vi "Generator.vi"() -> ()   [LabVIEW 2021]
uses:
  <vilib>/Utility/miscctls.llb/LV3DPointTypeDef.ctl
  <vilib>/picture/3D Picture Control/Object/Create Object (drawable).vi
  <vilib>/picture/3D Picture Control/Object/Add Object (no reference).vi
  <vilib>/picture/3D Picture Control/NI_3D Picture Control.lvlib
panel:
  in  "stop":bool
  out "Ball 2 Position":T1
  out "Ball 1 Position":T1
  out "Arm Base Position":T1
  in  "Z axis deg":sgl(slide) min=0 max=360 step=1 scale=0.0..360.0
  in  "Y axis deg":sgl(slide) min=0 max=360 step=1 scale=0.0..360.0
  in  "X Axis Degrees":sgl(slide) min=0 max=360 step=1 scale=0.0..360.0
  in  "X axis deg":sgl(slide) min=0 max=360 step=1 scale=0.0..360.0
  in  "Wall":dbl(slide)=0.5 min=0.0 max=1.0 step=0.05 scale=0.0..1.0
  in  "Background":u32(colorbox)=5789784
  in  "Axis Color":u32(colorbox)=16448250
  in  "Wall Color":u32(colorbox)=6618880
  in  "Machine Color":u32(colorbox)=16711680
  out "Test Area":refnum<vi>(3d-picture)
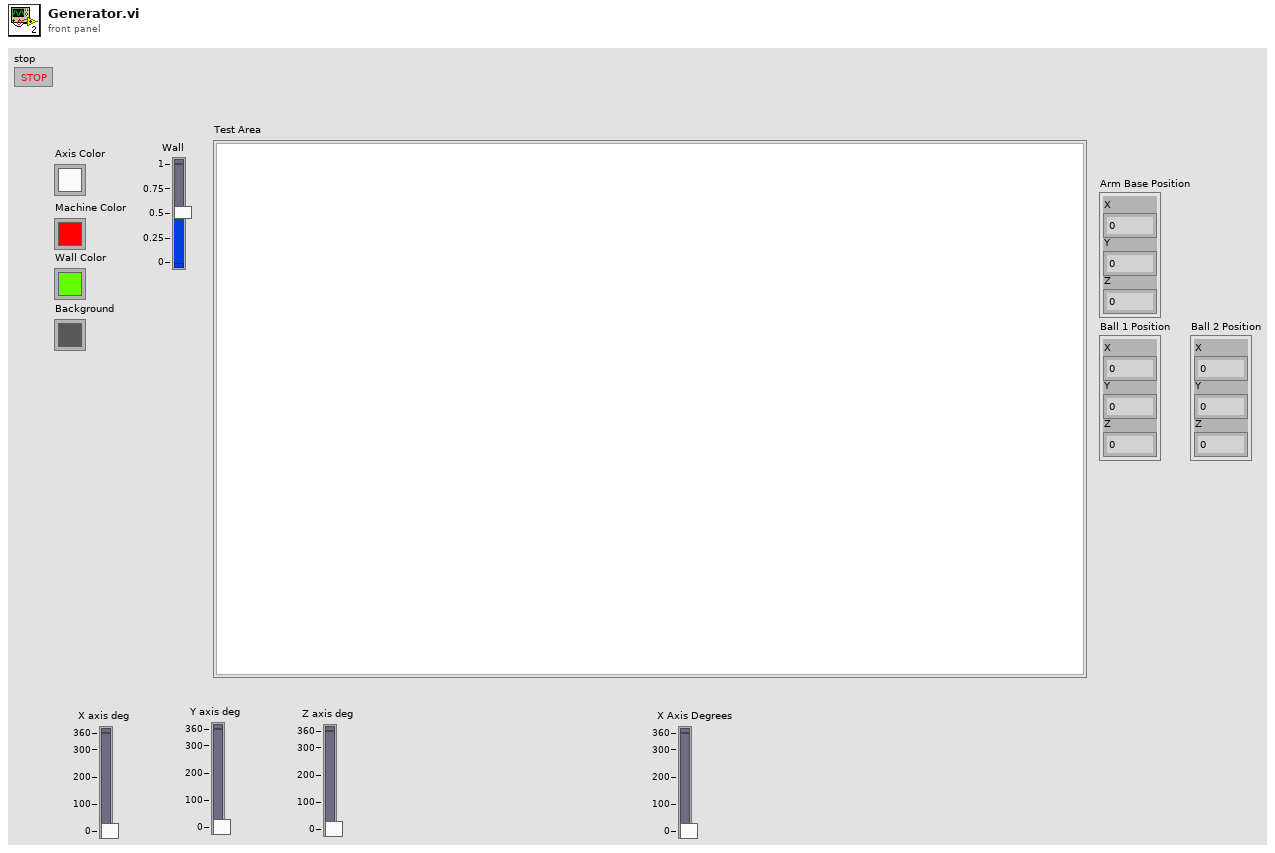
[diagram p1: front panel]
types:
  T1 = typedef "LV3DPointTypeDef.ctl" = cluster{"X":sgl, "Y":sgl, "Z":sgl}
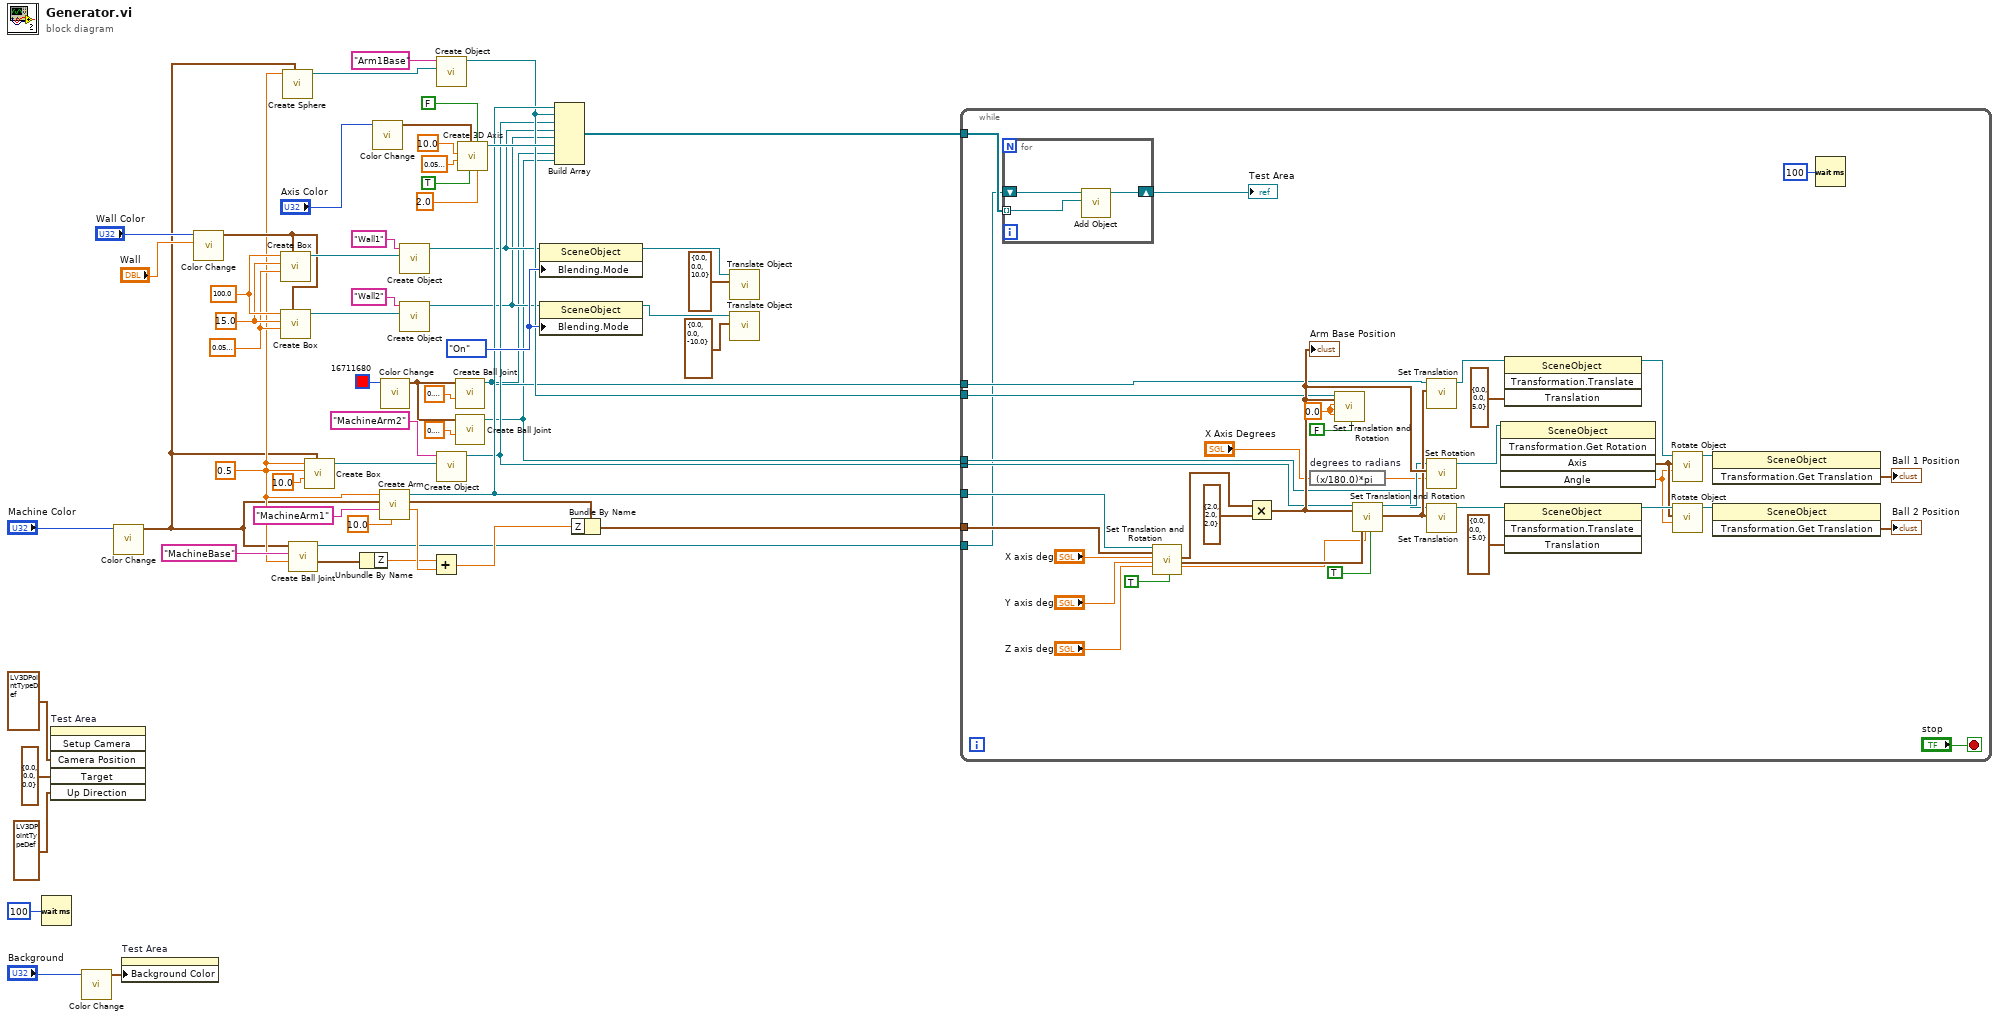
[diagram p0: block diagram]
diagram:
  w17 = sgl 0.5 ("Radius 2")
  w32 = enum16{"Inherit Value", "Off", "On"}."On" ("Blending:Mode")
  w47 = sgl 0.05 ("Length X")
  w48 = sgl 15.0 ("Length X")
  w49 = sgl 100.0 ("Length X")
  n1 = Wait (ms)(milliseconds to wait=u32 100) -> ()  [unwired: 1 out]
  n2 = invoke on="Test Area" class="SceneGraphDisp (strict)" method="Setup Camera"("Camera Position"=T1 {"X"=25.4, "Y"=40.2, "Z"=20.3}, "Target"=T1 {"X"=0.0, "Y"=0.0, "Z"=0.0}, "Up Direction"=T1 {"X"=0.2, "Y"=0.3, "Z"=0.4}) -> ()  [unwired: 3 in, 6 out]
  n3 = call <vilib>:"Color Change.vi"("Color"="Background") -> ("RGBA"=w38:cluster{"R":sgl, "G":sgl, "B":sgl, "A":sgl})  [unwired: 10 in]
  n4 = call <vilib>:"Color Change.vi"("Color"="Machine Color") -> ("RGBA"=w16:cluster{"R":sgl, "G":sgl, "B":sgl, "A":sgl})  [unwired: 10 in]
  n5 = property on="Test Area" class="SceneGraphDisp (strict)"("Background Color"=w38) -> ()  [unwired: 2 in, 2 out]
  n6 = call <vilib>:"Color Change.vi"("Alpha"="Wall", "Color"="Wall Color") -> ("RGBA"=w42:cluster{"R":sgl, "G":sgl, "B":sgl, "A":sgl})  [unwired: 9 in]
  n7 = call <vilib>:"Create Box.vi"("Color"=w42, "Length Z"=w47, "Length Y"=w48, "Length X"=w49) -> ("New Box Refnum"=w50:refnum<vi>)  [unwired: 6 in, 1 out]
  n8 = call <vilib>:"Create Box.vi"("Color"=w42, "Length Z"=w47, "Length Y"=w48, "Length X"=w49) -> ("New Box Refnum"=w34:refnum<vi>)  [unwired: 6 in, 1 out]
  n9 = call <vilib>:"Create Sphere.vi"("Color"=w16, "Radius"=w17) -> ("New Sphere Refnum"=w25:refnum<vi>)  [unwired: 8 in, 1 out]
  n10 = call "Create Ball Joint.vi"("Radius 2"=w17, "Name"="MachineBase", "RGBA"=w16) -> ("Transformation.GetTranslation"=w20:T1, "SceneObject out"=w1:refnum<vi>)  [unwired: 7 in]
  n11 = call <vilib>:"Create Box.vi"("Color"=w16, "Length Z"=sgl 10.0, "Length Y"=w17, "Length X"=w17) -> ("New Box Refnum"=w22:refnum<vi>)  [unwired: 6 in, 1 out]
  n12 = Unbundle By Name(w20) -> ("Z"=w19:sgl)
  n13 = call <vilib>:"Color Change.vi"("Color"="Axis Color") -> ("RGBA"=w40:cluster{"R":sgl, "G":sgl, "B":sgl, "A":sgl})  [unwired: 10 in]
  n14 = call "Create Arm.vi"("Length"=sgl 10.0 ("Length Z"), "Name"="MachineArm1", "Color"=w16, "Radius"=w17) -> ("Half Length"=w26:sgl, "Transformation.GetTranslation"=w30:T1, "SceneObject out"=w9:refnum<vi>)  [unwired: 5 in]
  n15 = call <vilib>:"Color Change.vi"("Color"=u32 16711680) -> ("RGBA"=w12:cluster{"R":sgl, "G":sgl, "B":sgl, "A":sgl})  [unwired: 10 in]
  n16 = call-poly <vilib>:"Create Object.vi"("Geometry"=w50, "Name"="Wall1") -> ("Scene:New Object"=w6:refnum<vi>)  [unwired: 8 in, 1 out]
  n17 = call-poly <vilib>:"Create Object.vi"("Geometry"=w34, "Name"="Wall2") -> ("Scene:New Object"=w5:refnum<vi>)  [unwired: 8 in, 1 out]
  n18 = Add(x=w19, y=w26) -> (x+y=w28:sgl)
  n19 = call-poly <vilib>:"Create Object.vi"("Geometry"=w25, "Name"="Arm1Base") -> ("Scene:New Object"=w8:refnum<vi>)  [unwired: 8 in, 1 out]
  n20 = call-poly <vilib>:"Create Object.vi"("Geometry"=w22, "Name"="MachineArm2") -> ("Scene:New Object"=w7:refnum<vi>)  [unwired: 8 in, 1 out]
  n21 = call "Create Ball Joint.vi"("Radius 2"=sgl 0.6, "RGBA"=w12) -> ("SceneObject out"=w4:refnum<vi>)  [unwired: 8 in, 1 out]
  n22 = call "Create Ball Joint.vi"("Radius 2"=sgl 0.6, "RGBA"=w12) -> ("SceneObject out"=w3:refnum<vi>)  [unwired: 8 in, 1 out]
  n23 = call <vilib>:"Create 3D Axis.vi"("Character Size"=sgl 2.0, "Half plane?"=FALSE, "Axis label?"=TRUE, "Color"=w40, "Radius"=sgl 0.05, "Length"=sgl 10.0) -> ("New Object Refnum"=w10:refnum<vi>)  [unwired: 4 in, 1 out]
  n24 = property class="SceneObject"(reference=w6, "Blending.Mode"=w32) -> (reference out=w35:refnum<vi>)  [unwired: 1 in, 1 out]
  n25 = property class="SceneObject"(reference=w5, "Blending.Mode"=w32) -> (reference out=w33:refnum<vi>)  [unwired: 1 in, 1 out]
  n26 = Build Array(w9, w8, w7, w6, w5, w10, w4, w3) -> (w2:refnum<vi>[])
  n27 = Bundle By Name(cluster=w30, "Z"=w28) -> (w29:T1)
  n28 = call <vilib>:"Translate Object.vi"("Translation"=cluster{"X":sgl, "Y":sgl, "Z":sgl} {"X"=0.0, "Y"=0.0, "Z"=10.0}, "Scene.Object In"=w35) -> ()  [unwired: 8 in, 2 out]
  n29 = call <vilib>:"Translate Object.vi"("Translation"=cluster{"X":sgl, "Y":sgl, "Z":sgl} {"X"=0.0, "Y"=0.0, "Z"=-10.0}, "Scene.Object In"=w33) -> ()  [unwired: 8 in, 2 out]
  n30 = while {
    tunnel: w29 -> [w99]
    tunnel: w9 -> [w69]
    tunnel: w8 -> [w68]
    tunnel: w7 -> [w67]
    tunnel: w4 -> [w66]
    tunnel: w3 -> [w65]
    tunnel: w2 -> [w63]
    tunnel: w1 -> [w62]
    stop <- "stop" stop-if-true
    w71 = sgl 0.0 ("X axis deg")
    n31 = for {
      tunnel: w63 -> [w101] mode=indexing
      shift-right: [w100] -> w61
      shift-left: w62 -> [w102]
      n32 = call-poly <vilib>:"Add Object.vi"("New Object In"=w101, "Scene Object In"=w102) -> ("Scene Object Out"=w100:refnum<vi>)  [unwired: 8 in, 1 out]
    }
    "Test Area" <- w61
    n33 = call "Set Translation and Rotation.vi"("SceneObject in"=w69, "Transformation.GetTranslation in"=w99, "X axis deg"="X axis deg", "Y axis deg"="Y axis deg", "Z axis deg"="Z axis deg", "Relative?"=TRUE) -> ("Transformation.GetTranslation out"=w94:T1, "Rotation Axis Out"=w92:T1, "Angle Out"=w89:sgl)  [unwired: 10 in, 1 out]
    n34 = Multiply(x=w94, y=T1 {"X"=2.0, "Y"=2.0, "Z"=2.0}) -> (x*y=w96:T1)
    "Arm Base Position" <- w96
    n35 = expression code="(x/180.0)*pi" "degrees to radians"("X Axis Degrees") -> (w73:sgl)
    n36 = call "Set Translation and Rotation.vi"("SceneObject in"=w68, "Transformation.GetTranslation in"=w96, "X axis deg"=w71, "Y axis deg"=w71, "Z axis deg"=w71, "Relative?"=FALSE) -> ()  [unwired: 10 in, 4 out]
    n37 = call "Set Translation and Rotation.vi"("SceneObject in"=w67, "Transformation.GetTranslation in"=w96, "Initial Rotation Axis"=w92, "Initial Rotation Angle"=w89, "Relative?"=TRUE) -> ("SceneObject out"=w74:refnum<vi>, "Transformation.GetTranslation out"=w80:T1)  [unwired: 11 in, 2 out]
    n38 = call <vilib>:"Set Translation.vi"("Translation"=w80, "Scene Object"=w66) -> ("Translated Object"=w88:refnum<vi>)  [unwired: 8 in, 1 out]
    n39 = call <vilib>:"Set Rotation.vi"("Angle"=w73, "Axis"=w96, "Scene Object"=w74) -> ("Rotated Scene Object"=w72:refnum<vi>)  [unwired: 7 in, 1 out]
    n40 = call <vilib>:"Set Translation.vi"("Translation"=w80, "Scene Object"=w65) -> ("Translated Object"=w83:refnum<vi>)  [unwired: 8 in, 1 out]
    n41 = invoke class="SceneObject" method="Transformation.Get Rotation"(reference=w72) -> ("Axis"=w82:T1, "Angle"=w81:sgl)  [unwired: 4 in, 3 out]
    n42 = invoke class="SceneObject" method="Transformation.Translate"(reference=w88, "Translation"=T1 {"X"=0.0, "Y"=0.0, "Z"=5.0} ("y")) -> (reference out=w86:refnum<vi>)  [unwired: 2 in, 3 out]
    n43 = invoke class="SceneObject" method="Transformation.Translate"(reference=w83, "Translation"=T1 {"X"=0.0, "Y"=0.0, "Z"=-5.0} ("y")) -> (reference out=w85:refnum<vi>)  [unwired: 2 in, 3 out]
    n44 = call <vilib>:"Rotate Object.vi"("Angle"=w81, "Axis"=w82, "Scene.Object In"=w86) -> ("Scene.Object Out"=w79:refnum<vi>)  [unwired: 7 in, 1 out]
    n45 = call <vilib>:"Rotate Object.vi"("Angle"=w81, "Axis"=w82, "Scene.Object In"=w85) -> ("Scene.Object Out"=w76:refnum<vi>)  [unwired: 7 in, 1 out]
    n46 = invoke class="SceneObject" method="Transformation.Get Translation"(reference=w79) -> ("Transformation.GetTranslation"=→"Ball 1 Position":T1)  [unwired: 2 in, 2 out]
    n47 = invoke class="SceneObject" method="Transformation.Get Translation"(reference=w76) -> ("Transformation.GetTranslation"=→"Ball 2 Position":T1)  [unwired: 2 in, 2 out]
    n48 = Wait (ms)(milliseconds to wait=u32 100) -> ()  [unwired: 1 out]
  }
